vi "Encoder-Decoder.vi"(10 "Encoder data":T1) -> (1 "Raw bits":bool[](array[boolean]), 2 "Converted bits":bool[](array[boolean]), 3 "Encoder position":u16)   [LabVIEW 2016]
doc: "Encoder-Decoder takes the 14 bits from the encoder which uses the Gray Protocol for encoding position information. The first element in the cluster is the Most Significant Bit (MSB) and the last element is the Least Significant Bit (LSB)"
uses:
  Encoder bit cluster.ctl
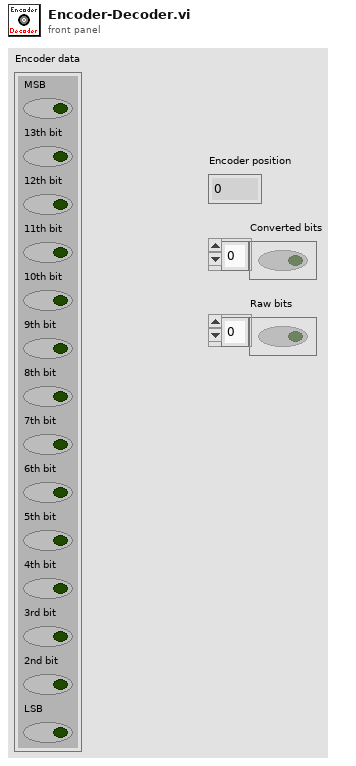
[diagram p1: front panel]
types:
  T1 = typedef "Encoder bit cluster.ctl" = cluster{"MSB":bool, "13th bit":bool, "12th bit":bool, "11th bit":bool, "10th bit":bool, "9th bit":bool, "8th bit":bool, "7th bit":bool, "6th bit":bool, "5th bit":bool, "4th bit":bool, "3rd bit":bool, "2nd bit":bool, "LSB":bool}
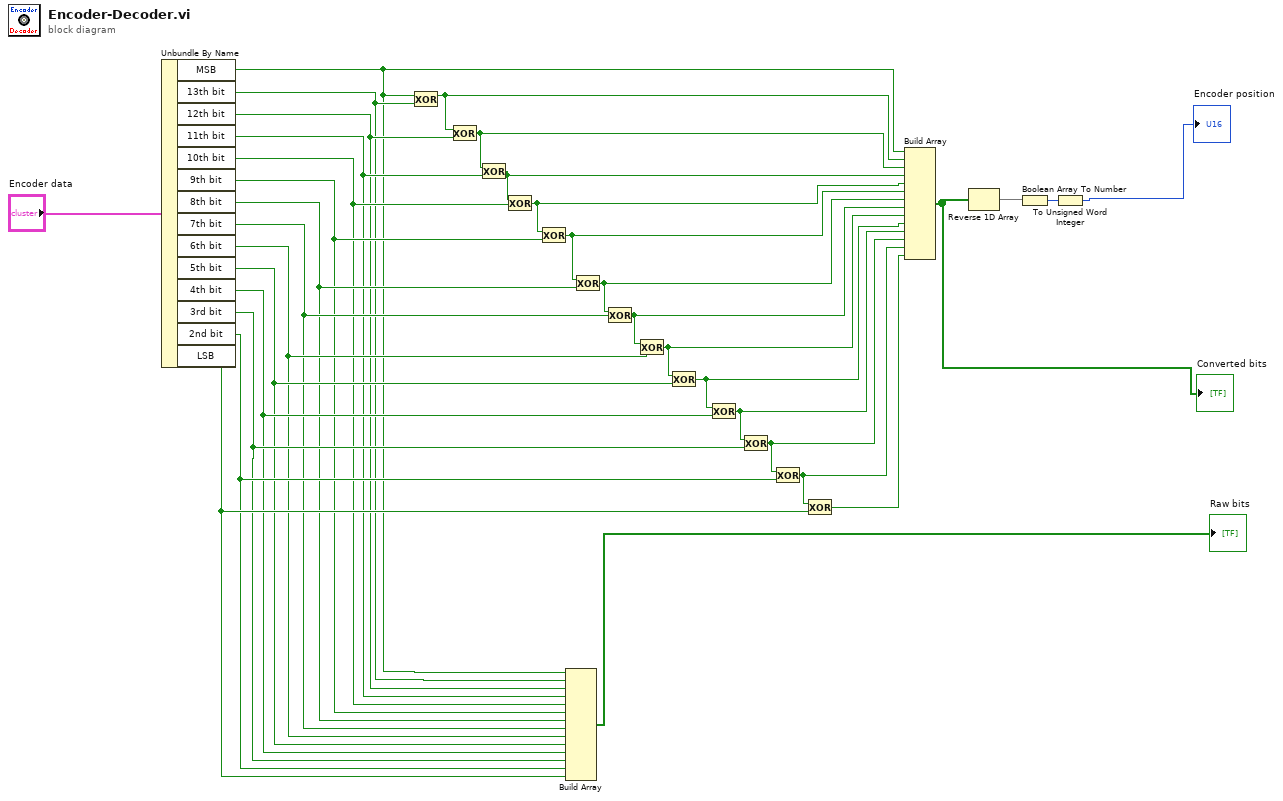
[diagram p0: block diagram]
diagram:
  n1 = Unbundle By Name("Encoder data") -> ("MSB"=w20:bool, "13th bit"=w21:bool, "12th bit"=w22:bool, "11th bit"=w23:bool, "10th bit"=w24:bool, "9th bit"=w25:bool, "8th bit"=w26:bool, "7th bit"=w27:bool, "6th bit"=w28:bool, "5th bit"=w29:bool, "4th bit"=w30:bool, "3rd bit"=w31:bool, "2nd bit"=w32:bool, "LSB"=w33:bool)
  n2 = Exclusive Or(1:w21, 2:w20) -> (0:w16:bool)
  n3 = Exclusive Or(1:w22, 2:w16) -> (0:w2:bool)
  n4 = Exclusive Or(1:w23, 2:w2) -> (0:w3:bool)
  n5 = Exclusive Or(1:w24, 2:w3) -> (0:w4:bool)
  n6 = Exclusive Or(1:w25, 2:w4) -> (0:w5:bool)
  n7 = Build Array(w20, w21, w22, w23, w24, w25, w26, w27, w28, w29, w30, w31, w32, w33) -> (→"Raw bits":bool[])
  n8 = Exclusive Or(1:w26, 2:w5) -> (0:w6:bool)
  n9 = Exclusive Or(1:w27, 2:w6) -> (0:w7:bool)
  n10 = Exclusive Or(1:w28, 2:w7) -> (0:w8:bool)
  n11 = Exclusive Or(1:w29, 2:w8) -> (0:w9:bool)
  n12 = Exclusive Or(1:w30, 2:w9) -> (0:w10:bool)
  n13 = Exclusive Or(1:w31, 2:w10) -> (0:w11:bool)
  n14 = Exclusive Or(1:w32, 2:w11) -> (0:w12:bool)
  n15 = Exclusive Or(1:w33, 2:w12) -> (0:w13:bool)
  n16 = Build Array(w20, w16, w2, w3, w4, w5, w6, w7, w8, w9, w10, w11, w12, w13) -> (w17:bool[])
  "Converted bits" <- w17
  n17 = Reverse 1D Array(array=w17) -> (reversed array=w14:bool[])
  n18 = Boolean Array To Number(Boolean array=w14) -> (number=w15:u32)
  n19 = To Unsigned Word Integer(number=w15) -> (unsigned 16bit integer=→"Encoder position":u16)
